vi "create error headers.vi"(10 "custom error reason":string, 11 "application request in":T1) -> (2 "values":string[](array[string]), 3 "fields":string[](array[string]))   [LabVIEW 2013, in "Basic HTTP server.lvclass"]
uses:
  Basic HTTP server.lvclass
  http request.ctl
  http method.ctl
  URI/url structure.ctl
  HTTP headers/http header data.ctl
  HTTP headers/http headers.lvlib
  URI/uniform resource locator.lvlib
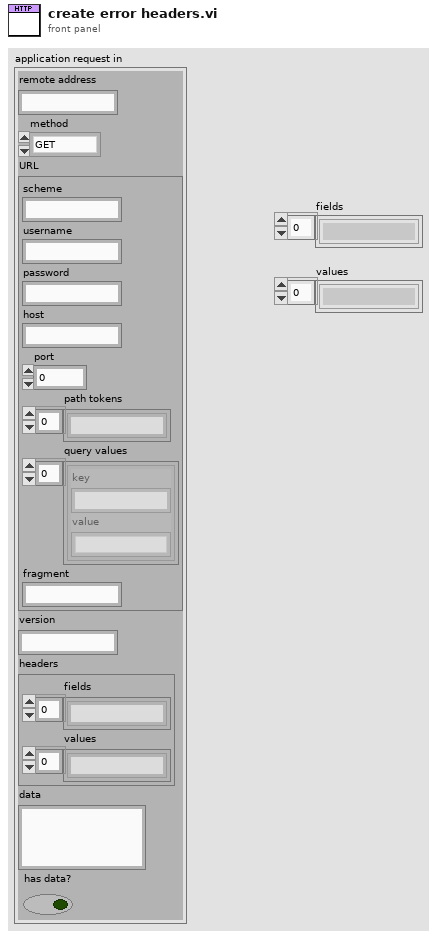
[diagram p1: front panel]
types:
  T1 = typedef "Basic HTTP server.lvclass/http request.ctl" = cluster{"remote address":string, "method":T2, "URL":T3, "version":string, "headers":T4, "data":string, "has data?":bool}
  T2 = typedef "Basic HTTP server.lvclass/http method.ctl" = enum16{"GET", "POST", "PUT", "DELETE", "HEAD", "OPTIONS", "upgrade"}
  T3 = typedef "uniform resource locator.lvlib/url structure.ctl" = cluster{"scheme":string, "username":string, "password":string, "host":string, "port":u16, "path tokens":string[], "query values":cluster{"key":string, "value":string}[], "fragment":string}
  T4 = typedef "http headers.lvlib/http header data.ctl" = cluster{"fields":string[], "values":string[]}
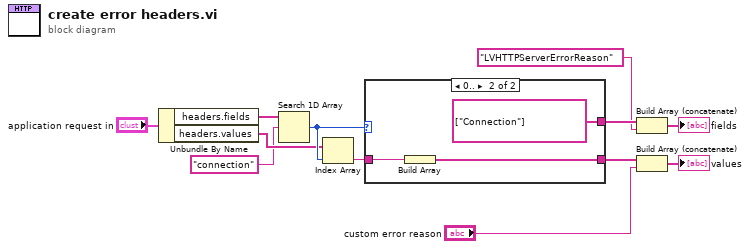
[diagram p0: block diagram]
diagram:
  n1 = Unbundle By Name("application request in") -> ("headers.fields"=w2:string[], "headers.values"=w4:string[])
  n2 = Search 1D Array(1D array=w2, element="connection" ("name")) -> (index of element=w5:i32)  [unwired: 1 in]
  n3 = Index Array(array=w4, index=w5) -> (element=w11:string)
  n4 = case shown="0.." w5 {
    tunnel: [_ w14] -> w10
    tunnel: w11 -> [_ w15]
    tunnel: [_ string[] ["Connection"]] -> w12
    frame ..-1 {
    }
    frame 0.. {
      n5 = Build Array(w15) -> (w14:string[])
    }
  }
  n6 = Build Array (concatenate)(w12, "LVHTTPServerErrorReason" ("error header")) -> (→"fields":string[])
  n7 = Build Array (concatenate)(w10, "custom error reason") -> (→"values":string[])
